vi "Add Signal Channel.vi"(6 "Signal Channel":variant, 9 "Signal Index":i32, 10 "QObject Refnum":u64, 11 "Signal Map":variant) -> (3 "Modified Signal Map":variant)   [LabVIEW 2013, in "Template.lvlib" / "LQWidgetEngine.lvclass"]
uses:
  LQWidgetEngine.lvclass
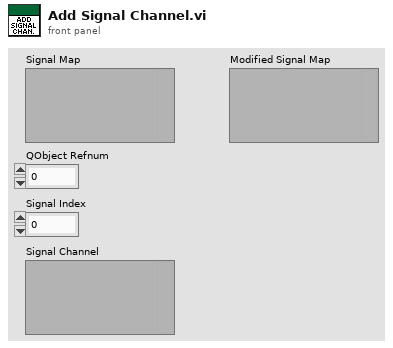
[diagram p1: front panel]
types:
  T1 = enum16{"big-endian, network order", "native, host order", "little-endian"}
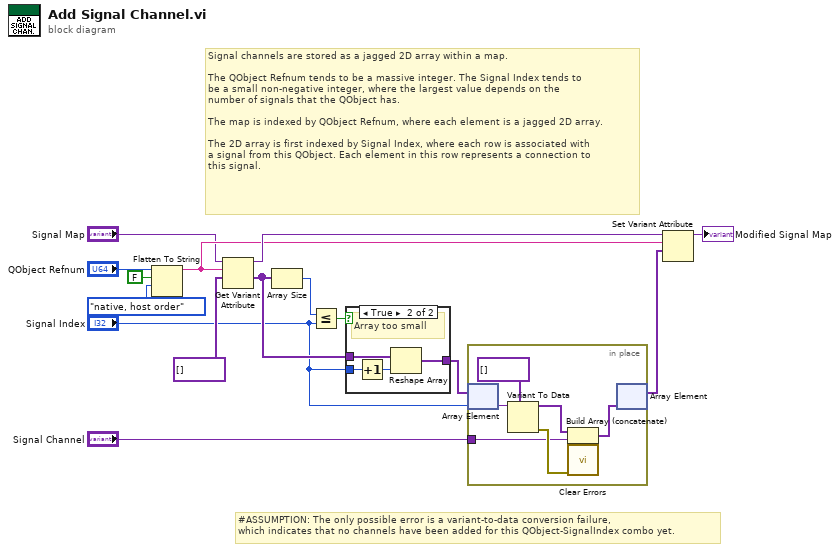
[diagram p0: block diagram]
diagram:
  # "Signal channels are stored as a jagged 2D array within a map.\n\nThe QObject Refnum tends to be a massive integer. The Signal Index tends to\nbe a small non-negative integer, where the largest value depends on the\nnumber of signals that the QObject has.\n\nThe map is indexed by QObject Refnum, where each element is a jagged 2D array.\n\nThe 2D array is first indexed by Signal Index, where each row is associated with\na signal from this QObject. Each element in this row represents a connection to\nthis signal."
  # "#ASSUMPTION: The only possible error is a variant-to-data conversion failure,\nwhich indicates that no channels have been added for this QObject-SignalIndex combo yet."
  n1 = Flatten To String(anything="QObject Refnum", prepend array or string size? (T)=FALSE, byte order (0:big-endian, network order)=T1."native, host order") -> (data string=w9:string)  [unwired: 1 in, 2 out]
  n2 = Get Variant Attribute(Variant="Signal Map", name=w9, default value (empty Variant)=variant[] []) -> (duplicate Variant=w10:variant, value=w13:variant[])  [unwired: 1 in, 2 out]
  n3 = Array Size(array=w13) -> (size(s)=w12:i32)
  n4 = Less Or Equal?(x=w12, y="Signal Index") -> (x <= y?=w11:bool)
  n5 = case shown="True" w11 {
    tunnel: w13 -> [w16 w20]
    tunnel: "Signal Index" -> [_ w19]
    tunnel: [w16 w17] -> w7
    frame False {
      # "It fits"
    }
    frame True {
      # "Array too small"
      n6 = Increment(x=w19) -> (x+1=w18:i32)
      n7 = Reshape Array(w20, w18) -> (w17:variant[])
    }
  }
  n8 = in-place {
    in-place-border: "Signal Channel" -> [w23]
    n9 = in-place-array #1(w7, "Signal Index") -> (w24:variant)
    n10 = Variant To Data(type=variant[] [], Variant=w24) -> (data=w25:variant[], error out=w26:errorcluster)  [unwired: 1 in]
    n11 = Build Array (concatenate)(w25, w23) -> (w22:variant[])
    n12 = call <vilib>:"Clear Errors.vi"("error in (no error)"=w26) -> ()  [unwired: 6 in, 1 out]
    n13 = in-place-array #1(w22) -> (w6:variant[])  [unwired: 1 out]
  }
  n14 = Set Variant Attribute(Variant=w10, name=w9, value=w6) -> (Variant out=→"Modified Signal Map":variant)  [unwired: 1 in, 2 out]
